vi "Create MetaData Channel - Single Channel - Type Cast.vi"(8 "Error In":errorcluster, 9 "Settings":T1, 10 "Name":string, 11 "Message Refnum In":T4=18446744073709551615 format="%.0x") -> (0 "Error Out":errorcluster, 2 "Channel Refnum":T4=18446744073709551615 format="%.0x", 3 "Message Refnum Out":T4=18446744073709551615 format="%.0x")   [LabVIEW 2018, in "Instrument Addon Scripting API.lvlib"]
uses:
  Instrument Addon Scripting API.lvlib
  <vilib>/NI Veristand/Custom Device API/Custom Device Item Ref.ctl
  TypeDefs/Single Channel Type Cast Settings.ctl
  Addon/Addon Shared/Types/Type Cast Type.ctl
  Addon/Addon Shared/Types/Endian.ctl
  Addon/Addon Shared/Types/MetaData Parameters.ctl
  Addon/Addon Shared/Types/Protocol Data Type.ctl
  Addon/Addon Shared/Types/Metadata Channel Type.ctl
  TypeDefs/Channel Properties.ctl
  TypeDefs/MetaData Type.ctl
  Addon/Addon Shared/Instrument Addon Shared.lvlib
  <vilib>/NI Veristand/Custom Device API/Custom Device API.lvlib
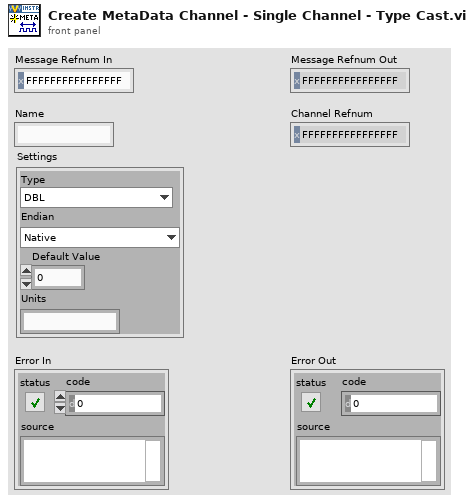
[diagram p1: front panel]
types:
  T1 = typedef "Instrument Addon Scripting API.lvlib/Single Channel Type Cast Settings.ctl" = cluster{"Type":T2, "Endian":T3, "Default Value":dbl, "Units":string}
  T2 = typedef "Instrument Addon Shared.lvlib/Type Cast Type.ctl" = enum16{"DBL", "SGL", "U64", "U32", "U16", "U8", "I64", "I32", "I16", "I8"}
  T3 = typedef "Instrument Addon Shared.lvlib/Endian.ctl" = enum16{"Native", "Little", "Big"}
  T4 = typedef "Custom Device API.lvlib/Custom Device Item Ref.ctl" = u64
  T5 = typedef "Instrument Addon Scripting API.lvlib/MetaData Type.ctl" = enum16{"MetaData", "Global MetaData"}
  T6 = typedef "Instrument Addon Scripting API.lvlib/Channel Properties.ctl" = cluster{"Default Value":dbl, "Units":string}
  T7 = typedef "Instrument Addon Shared.lvlib/Metadata Channel Type.ctl" = enum16{"Enumerated List", "Format", "Type Cast"}
  T8 = typedef "Instrument Addon Shared.lvlib/Protocol Data Type.ctl" = enum16{"Single Channel", "Array"}
  T9 = typedef "Instrument Addon Shared.lvlib/MetaData Parameters.ctl" = cluster{"Data Type":T8, "Channel Type":T7, "List":string[], "Format String":string, "Type":T2, "Delimiter":string, "Endian":T3}
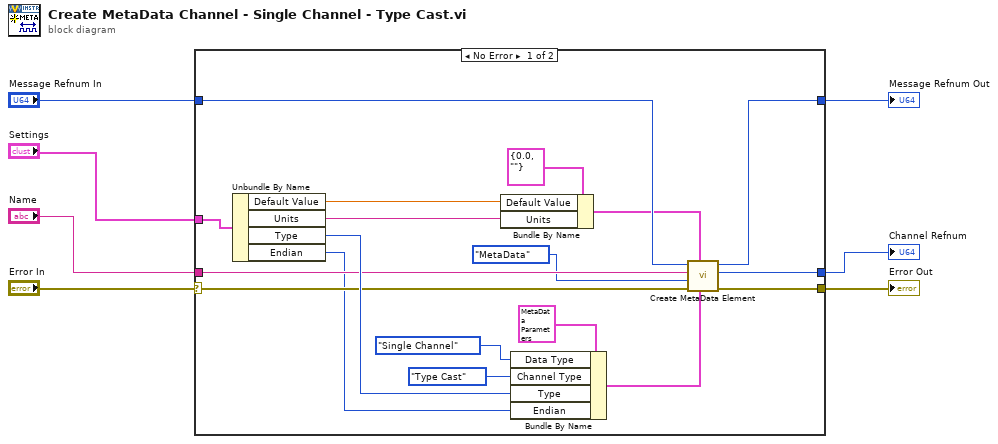
[diagram p0: block diagram]
diagram:
  n1 = case shown="No Error" "Error In" {
    selector: "Error In" -> [w10 w26]
    tunnel: [w25 w26] -> w7
    tunnel: "Settings" -> [w24 _]
    tunnel: "Message Refnum In" -> [w18 w27]
    tunnel: [w13 _] -> w5
    tunnel: [w12 w27] -> w4
    tunnel: "Name" -> [w11 _]
    frame No Error {
      n2 = Unbundle By Name(w24) -> ("Default Value"=w17:dbl, "Units"=w16:string, "Type"=w20:T2, "Endian"=w9:T3)
      n3 = Bundle By Name(cluster=T6 {"Default Value"=0.0, "Units"=""}, "Default Value"=w17, "Units"=w16) -> (w14:T6)
      n4 = Bundle By Name(cluster=T9 {"Data Type"=enum."Single Channel", "Channel Type"=enum."Format", "List"=[], "Format String"="%.3g", "Type"=enum."SGL", "Delimiter"="", "Endian"=enum."Native"} ("MetaData Parameters"), "Data Type"=Protocol_Data_Type."Single Channel", "Channel Type"=Metadata_Channel_Type."Type Cast", "Type"=w20, "Endian"=w9) -> (w19:T9)
      n5 = call "Create MetaData Element.vi"("MetaData Parameters"=w19, "Channel Properties"=w14, "error in (no error)"=w10, "Type"=MetaData_Type."MetaData", "Name"=w11, "Refnum In"=w18) -> ("error out"=w25:errorcluster, "Channel Refnum"=w13:T4, "Refnum Out"=w12:T4)  [unwired: 3 in]
    }
    frame Error {
    }
  }
  "Message Refnum Out" <- w4
  "Error Out" <- w7
  "Channel Refnum" <- w5
